vi "Write Shunt dU.vi"(8 "error in (no error)":errorcluster, 10 "Shunt dU":dbl caption="Heater I", 11 "LNG Boiling Results in":refnum<class "LNG Boiling Results.lvclass">) -> (0 "error out":errorcluster, 3 "LNG Boiling Results out":refnum<class "LNG Boiling Results.lvclass">)   [LabVIEW 2019, in "Results.lvlib" / "LNG Boiling Results.lvclass"]
uses:
  LNG Boiling Results.lvclass
  LNG Boiling Results.lvclass/LNG Boiling Results.ctl
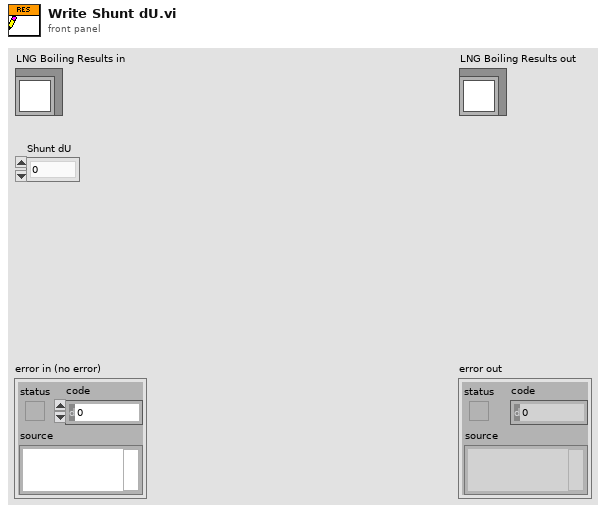
[diagram p1: front panel]
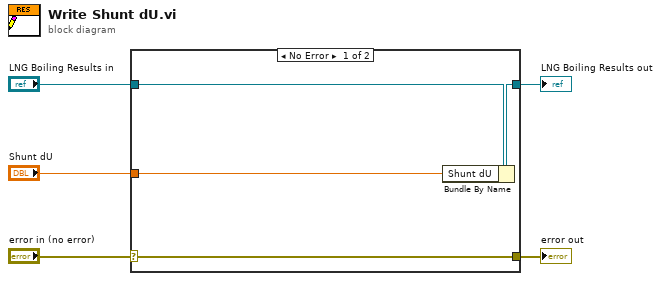
[diagram p0: block diagram]
diagram:
  n1 = case shown="No Error" "error in (no error)" {
    selector: "error in (no error)" -> [w9 w10]
    tunnel: [w9 w10] -> w4
    tunnel: [w7 w11] -> w2
    tunnel: "LNG Boiling Results in" -> [w8 w11]
    tunnel: "Shunt dU" -> [w6 _]
    frame No Error {
      n2 = Bundle By Name(cluster=w8, "Shunt dU"=w6) -> (w7:refnum<class "LNG Boiling Results.lvclass">)
    }
    frame Error {
    }
  }
  "error out" <- w4
  "LNG Boiling Results out" <- w2
